vi "Create Evaluation String.vi"(8 "error in (no error)":errorcluster, 10 "Evaluation String":string, 11 "Str Contains in":refnum<class "Str Contains.lvclass">) -> (0 "error out":errorcluster, 3 "Str Contains out":refnum<class "Str Contains.lvclass">)   [LabVIEW 2018, in "Str Contains.lvclass"]
uses:
  Str Contains.lvclass
  C:/Users/UKHornP/Documents/Work/Projects/Assert_API/Plugins/Utility/Test Classes/Test.lvclass
  String.lvclass
  Test.lvclass
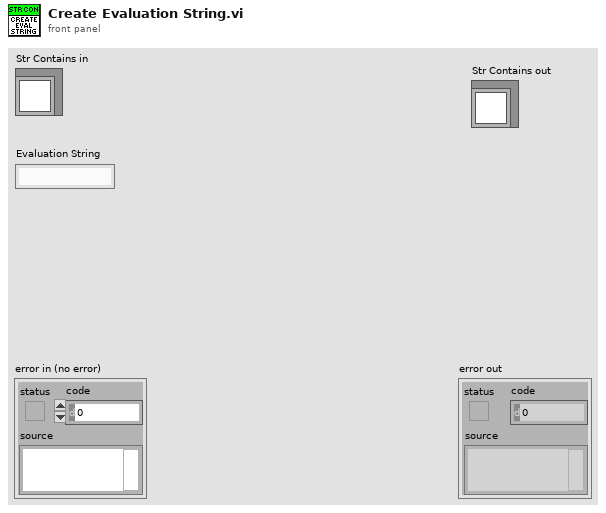
[diagram p1: front panel]
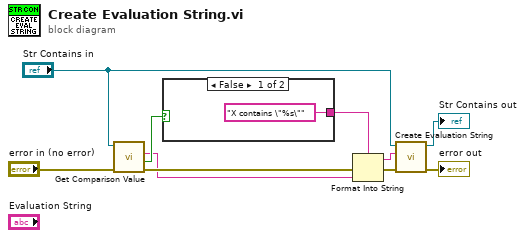
[diagram p0: block diagram]
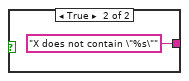
[diagram p2: hidden frame]
diagram:
  n1 = call "Get Comparison Value.vi"("error in (no error)"="error in (no error)", "Test in"="Str Contains in") -> ("error out"=w7:errorcluster, "Invert Result"=w4:bool, "Data String"=w2:string)  [unwired: 7 in]
  n2 = case shown="False" w4 {
    tunnel: ["X contains \"%s\"" "X does not contain \"%s\""] -> w3
    frame False {
    }
    frame True {
    }
  }
  n3 = Format Into String(format string=w3, error in=w7, w2) -> (resulting string=w1:string, error out=w5:errorcluster)  [unwired: 1 in]
  n4 = call-parent "Create Evaluation String.vi"("error in (no error)"=w5, "Evaluation String"=w1, "String in"="Str Contains in") -> ("error out"=→"error out":errorcluster, "String out"=→"Str Contains out":refnum<class "Str Contains.lvclass">)  [unwired: 7 in]
